vi "ROSServiceClient.vi"(2 "Response":T2, 3 "ROS":T3={"topic port"=1236, "Node"="/labview", "topic"="/robot/head/command_head_nod", "type"="std_msgs/Bool", "node port"=7000, "error "={"status"=FALSE, "code"=0, "source"=""}, "Direction"=enum."Publisher", "Update (ms)"=1, "FIFO size"=1}) -> ()   [LabVIEW 2012]
doc: "Opens new ports for services, updates services with master, and closes services"
uses:
  <userlib>/ROS for LabVIEW Software/ROS/Code/SubVIs/_ROSControl.ctl
  <userlib>/ROS for LabVIEW Software/ROS/Code/SubVIs/_ROSDirection.ctl
  <userlib>/ROS for LabVIEW Software/ROS/Code/Console/Servers/ServerSubs/MyState.ctl
  <userlib>/ROS for LabVIEW Software/ROS/Code/_ROSDefinition.vi
panel:
  out "Hex  Reply":string
  out "Queue log":string
  out "Listing":T1(array[cluster])
  out "Success?":bool
  out "Reply":string
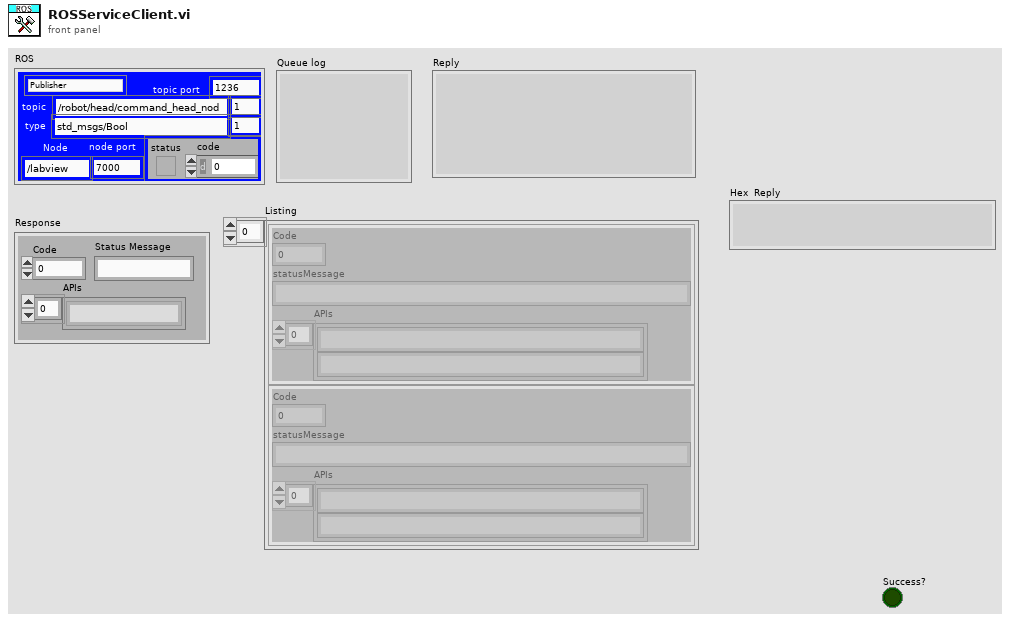
[diagram p1: front panel]
types:
  T1 = cluster{"Code":i8, "statusMessage":string, "APIs":string[]}[]
  T2 = cluster{"Code":i32, "Status Message":string, "APIs":string[]}
  T3 = typedef "_ROSControl.ctl" = cluster{"topic port":u16, "Node":string, "topic":string, "type":string, "node port":u16, "error ":errorcluster, "Direction":T4, "Update (ms)":u16, "FIFO size":u16}
  T4 = typedef "_ROSDirection.ctl" = enum16{"Node", "Publisher", "Subscriber", "ServiceClient", "ServiceProvider"}
  T5 = typedef "MyState.ctl" = enum16{"No Connection", "Registered", "Connected", "Close"}
  T6 = enum16{"Reset Log", "Add Client", "Remove Client", "Add Task"}
  T7 = typedef "ROSLog.ctl" = cluster{"Sent":string, "Reply":string, "MethodName":string, "success":bool, "Dir1":string, "Dir2":string, "Time Stamp":string, "error":errorcluster, "Preamble":string, "Midamble":string, "Postamble":string}
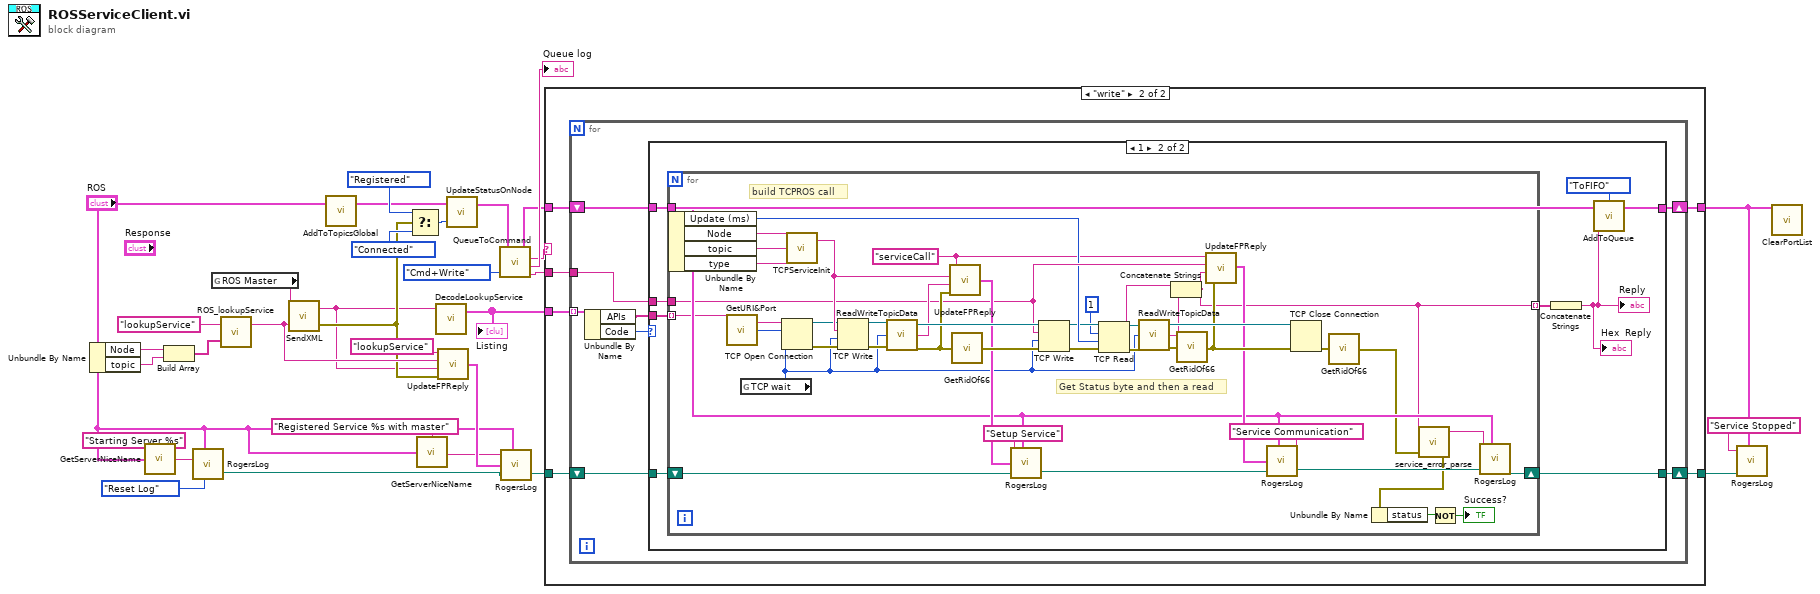
[diagram p0: block diagram]
diagram:
  n1 = Unbundle By Name("ROS") -> ("Node"=w29:string, "topic"=w28:string)
  n2 = call <userlib>:"GetServerNiceName.vi"("ROS"="ROS", "Text to add"="Starting Server %s") -> ("String"=w31:string)
  n3 = Build Array(w29, w28) -> (w27:string[])
  n4 = call <userlib>:"RogersLog.vi"("Text to add"=w31, "ROS"="ROS", "Task"=T6."Reset Log") -> ("LogPath out"=w18:path)  [unwired: 2 in, 1 out]
  n5 = global read "_ROSDefinition.vi" "ROS Master"() -> (w23:string)
  n6 = call <userlib>:"ROS_lookupService.vi"("Parameters"=w27, "Method Name"="lookupService") -> ("lookupService"=w25:string)  [unwired: 1 in]
  n7 = call <userlib>:"SendXML.vi"("Send"=w25, "URI in"=w23) -> ("error out"=w15:errorcluster, "Reply"=w14:string)
  n8 = call <userlib>:"AddToTopicsGlobal.vi"("ROS in"="ROS") -> ("ROS out"=w3:T3)  [unwired: 2 in]
  n9 = Select(t=MyState."Registered" ("MyState"), s=w15, f=MyState."Connected" ("MyState")) -> (s? t:f=w20:T5)
  n10 = call <userlib>:"GetServerNiceName.vi"("ROS"="ROS", "Text to add"="Registered Service %s with master") -> ("String"=w16:string)
  n11 = call <userlib>:"DecodeLookupService.vi"("Response"=w14) -> ("Reply"=w13:T1)  [unwired: 2 in]
  "Listing" <- w13
  n12 = call <userlib>:"UpdateFPReply.vi"("error in (no error)"=w15, "Reply"=w14, "Sent"=w25, "method"="lookupService" ("Method Name")) -> ("Log"=w19:T7)
  n13 = call <userlib>:"UpdateStatusOnNode.vi"("MyState"=w20, "ROS"=w3) -> ("ROS out"=w5:T3)  [unwired: 1 in]
  n14 = call <userlib>:"QueueToCommand.vi"("ROS"=w5, "Check"=enum16{"Cmd+Write", "FIFO", "CMD", "CMD /wait"}."Cmd+Write") -> ("ROS out"=w6:T3, "Command"=w1:string, "Queue log"=→"Queue log":string, "data"=w9:string)  [unwired: 1 in]
  n15 = call <userlib>:"RogersLog.vi"("Text to add"=w16, "ROS"="ROS", "Log"=w19, "LogPath in"=w18) -> ("LogPath out"=w11:path)  [unwired: 1 in, 1 out]
  n16 = case shown="\"write\"" w1 {
    tunnel: w13 -> [_ w39]
    tunnel: w6 -> [w33 w35]
    tunnel: w11 -> [w34 w38]
    tunnel: [w34 w37] -> w10
    tunnel: w9 -> [_ w36]
    tunnel: [w33 w35] -> w2
    frame Default {
    }
    frame "write" {
      n17 = for {
        tunnel: w39 -> [w47] mode=indexing
        shift-right: [w42] -> w37
        shift-left: w38 -> [w43]
        tunnel: w36 -> [w41]
        shift-right: [w40] -> _
        shift-left: w35 -> [w44]
        n18 = Unbundle By Name(w47) -> ("APIs"=w46:string[], "Code"=w45:i8)
        n19 = case shown="1" w45 {
          tunnel: w46 -> [_ w58]
          tunnel: w44 -> [w48 w52]
          tunnel: w43 -> [w49 w57]
          tunnel: [w49 w56] -> w42
          tunnel: w41 -> [_ w54]
          tunnel: [w48 w50] -> w40
          frame Default {
          }
          frame 1 {
            n20 = for {
              tunnel: w58 -> [w69] mode=indexing
              tunnel: w52 -> [w81]
              tunnel: [w77] -> w55 mode=indexing
              shift-right: [w75] -> w56
              shift-left: w57 -> [w76]
              tunnel: w54 -> [w74]
              w68 = "serviceCall" ("APIs")
              # "Get Status byte and then a read"
              # "build TCPROS call"
              n21 = Unbundle By Name(w81) -> ("Update (ms)"=w71:u16, "Node"=w80:string, "topic"=w79:string, "type"=w96:string)
              n22 = call <userlib>:"GetURI&Port.vi"("URI in"=w69) -> ("Port"=w103:u16, "URI"=w102:string)
              n23 = global read "_ROSDefinition.vi" "TCP wait"() -> (w59:i32)
              n24 = TCP Open Connection(address=w102, remote port or service name=w103, timeout ms (60000)=w59) -> (connection ID=w82:refnum<k5>, error out=w78:errorcluster)  [unwired: 2 in]
              n25 = call <userlib>:"TCPServiceInit.vi"("Type"=w96, "topic"=w79, "callerID"=w80) -> ("TCP ROS Reply"=w90:string)  [unwired: 1 in]
              n26 = TCP Write(connection ID=w82, data in=w90, error in (no error)=w78, 9:w59) -> (connection ID out=w101:refnum<k5>, error out=w100:errorcluster)  [unwired: 1 out]
              n27 = call <userlib>:"ReadWriteTopicData.vi"("error in (no error)"=w100, "timeout ms (1000)"=w59, "connection ID in"=w101) -> ("error out"=w85:errorcluster, "data out"=w89:string, "connection ID out"=w99:refnum<k5>)
              n28 = call <userlib>:"UpdateFPReply.vi"("error in (no error)"=w85, "Reply"=w89, "Sent"=w90, "method"=w68) -> ("Log"=w87:T7)
              n29 = call <userlib>:"GetRidOf66.vi"("error in (no error)"=w85) -> ("error out"=w88:errorcluster)
              n30 = call <userlib>:"RogersLog.vi"("Text to add"="Setup Service", "ROS"=w81, "Log"=w87, "LogPath in"=w76) -> ("LogPath out"=w94:path)  [unwired: 1 in, 1 out]
              n31 = TCP Write(connection ID=w99, data in=w74, error in (no error)=w88, 9:w59) -> (connection ID out=w66:refnum<k5>, error out=w65:errorcluster)  [unwired: 1 out]
              n32 = TCP Read(connection ID=w66, bytes to read=1, error in (no error)=w65, 9:w71) -> (connection ID out=w62:refnum<k5>, data out=w61:string, error out=w64:errorcluster)  [unwired: 1 in]
              n33 = call <userlib>:"ReadWriteTopicData.vi"("error in (no error)"=w64, "timeout ms (1000)"=w59, "connection ID in"=w62) -> ("error out"=w67:errorcluster, "data out"=w60:string, "connection ID out"=w98:refnum<k5>)
              n34 = Concatenate Strings(w61, w60) -> (w77:string)
              n35 = call <userlib>:"GetRidOf66.vi"("error in (no error)"=w67) -> ("error out"=w97:errorcluster)
              n36 = call <userlib>:"UpdateFPReply.vi"("error in (no error)"=w97, "Reply"=w77, "Sent"=w74, "method"=w68) -> ("Log"=w93:T7)
              n37 = call <userlib>:"RogersLog.vi"("Text to add"="Service Communication", "ROS"=w81, "Log"=w93, "LogPath in"=w94) -> ("LogPath out"=w84:path)  [unwired: 1 in, 1 out]
              n38 = TCP Close Connection(connection ID=w98, error in (no error)=w97) -> (error out=w83:errorcluster)  [unwired: 1 in, 1 out]
              n39 = call <userlib>:"GetRidOf66.vi"("error in (no error)"=w83) -> ("error out"=w73:errorcluster)
              n40 = call <userlib>:"service_error_parse.vi"("error in (no error)"=w73, "Reply"=w77) -> ("error out"=w72:errorcluster, "Log string"=w70:string)  [unwired: 1 in, 1 out]
              n41 = Unbundle By Name(w72) -> ("status"=w92:bool)
              n42 = Not(x=w92) -> (.not. x?=→"Success?":bool)
              n43 = call <userlib>:"RogersLog.vi"("Text to add"=w70, "ROS"=w81, "LogPath in"=w84) -> ("LogPath out"=w75:path)  [unwired: 2 in, 1 out]
            }
            n44 = Concatenate Strings(w55) -> (w51:string)
            "Reply" <- w51
            "Hex  Reply" <- w51
            n45 = call <userlib>:"AddToQueue.vi"("Cmd"=w51, "ROS"=w52, "Type"=enum16{"topic", "node", "ToFIFO"}."ToFIFO") -> ("ROS out"=w50:T3)  [unwired: 2 in]
          }
        }
      }
    }
  }
  n46 = call <userlib>:"RogersLog.vi"("Text to add"="Service Stopped", "ROS"=w2, "LogPath in"=w10) -> ()  [unwired: 2 in, 2 out]
  n47 = call <userlib>:"ClearPortList.vi"("ROS"=w2) -> ()  [unwired: 2 in]
